vi "Remove Comments from Single-line.vi"(3 "single-line text":string) -> (1 "single-line text without comments":string)   [LabVIEW 2017, in "CSM Shared.lvlib"]
uses:
  CSM Shared.lvlib
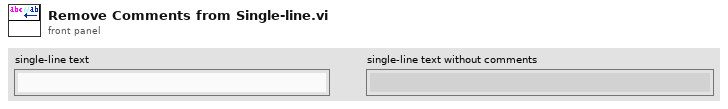
[diagram p1: front panel]
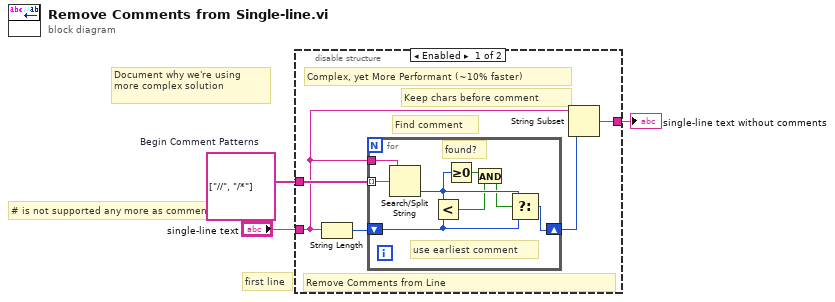
[diagram p0: block diagram]
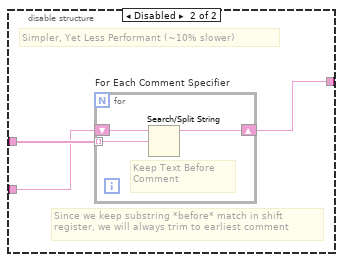
[diagram p2: hidden frame]
diagram:
  w3 = string[] ["//", "/*"]  # Begin Comment Patterns
  # "# is not supported any more as comment."
  # "Document why we're using more complex solution"
  # "first line"
  n1 = disable-structure "Diagram Disable Structure" shown="Enabled" {
    disable-tunnel: w3 -> [w8 w19]
    disable-tunnel: [w7 w18] -> w1
    disable-tunnel: "single-line text" -> [w6 w17]
    frame Enabled {
      # "Remove Comments from Line"
      # "Complex, yet More Performant (~10% faster)"
      # "Keep chars before comment"
      # "Find comment"
      n2 = String Length(string=w6) -> (length=w5:i32)
      n3 = for {
        tunnel: w8 -> [w13] mode=indexing
        shift-right: [w15] -> w4
        shift-left: w5 -> [w16]
        tunnel: w6 -> [w14]
        # "found?"
        # "use earliest comment"
        n4 = Search/Split String(string=w14, search string/char (-)=w13) -> (offset of match=w12:i32)  [unwired: 1 in, 2 out]
        n5 = Less?(x=w12, y=w16) -> (x < y?=w10:bool)
        n6 = Greater Or Equal To 0?(x=w12) -> (x >= 0?=w11:bool)
        n7 = And(x=w11, y=w10) -> (x .and. y?=w9:bool)
        n8 = Select(t=w12, s=w9, f=w16) -> (s? t:f=w15:i32)
      }
      n9 = String Subset(string=w6, length (rest)=w4) -> (substring=w7:string)  [unwired: 1 in]
    }
    frame Disabled {
      # "Since we keep substring *before* match in shift register, we will always trim to earliest comment"
      # "Simpler, Yet Less Performant (~10% slower)"
      n10 = for "For Each Comment Specifier" {
        tunnel: w19 -> [w21] mode=indexing
        shift-right: [w20] -> w18
        shift-left: w17 -> [w22]
        # "Keep Text Before Comment"
        n11 = Search/Split String(string=w22, search string/char (-)=w21) -> (substring before match=w20:string)  [unwired: 1 in, 2 out]
      }
    }
  }
  "single-line text without comments" <- w1
